vi "Retrieve Data.vi"(8 "error in (no error)":errorcluster, 11 "Vaisala in":refnum<class "FPGA Vaisala.lvclass">) -> (0 "error out":errorcluster, 2 "Str Out":string, 3 "Vaisala out":refnum<class "FPGA Vaisala.lvclass">)   [LabVIEW 2014, in "FPGA Vaisala.lvclass"]
uses:
  FPGA Vaisala.lvclass
  <vilib>/rvi/interface/nirviReadWriteControl/nirviReadWriteControl.xnode
  <vilib>/rvi/errors/niLvFpgaAdjustHostInterfaceError.vi
  Instruments/Nicholas/FPGA/RS485 In.ctl
  <vilib>/rvi/interface/nirviMethod/nirviMethod.xnode
  <vilib>/rvi/errors/niLvFpgaMergeErrorWithErrorCode.vi
  <vilib>/FPGAPlugInAG/cRIO-9081/niLvFpga_AcknowledgeIrq_cRIO-9081.vi
  <vilib>/rvi/interface/nirviMethod/StockFPGA_InlinedMethodWaitForSingleIRQ.vi
  <vilib>/FPGAPlugInAG/cRIO-9081/niLvFpga_WaitOnIrq_cRIO-9081.vi
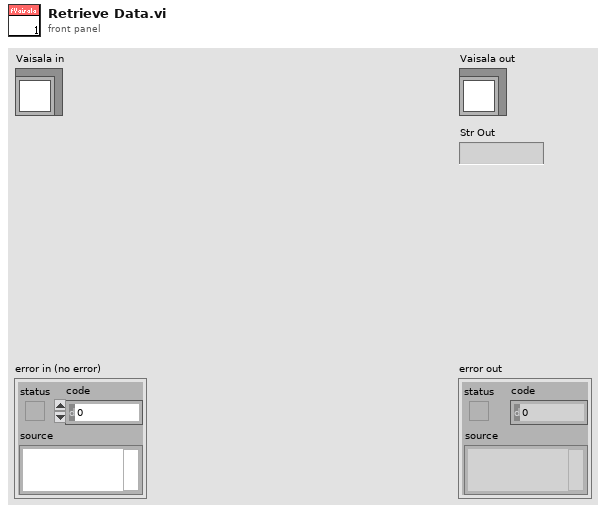
[diagram p1: front panel]
types:
  T1 = typedef "RS485 In.ctl" = cluster{"Data":u8[], "NumBytes":i32, "RS485_Cmd":enum16{"Read", "Write", "Idle"}, "New":bool, "Port":enum16{"Port 1", "Port 2", "Port 3", "Port 4", "None"}, "Timeout (ms)":i32}
  T2 = enum16{"Port 1", "Port 2", "Port 3", "Port 4", "None"}
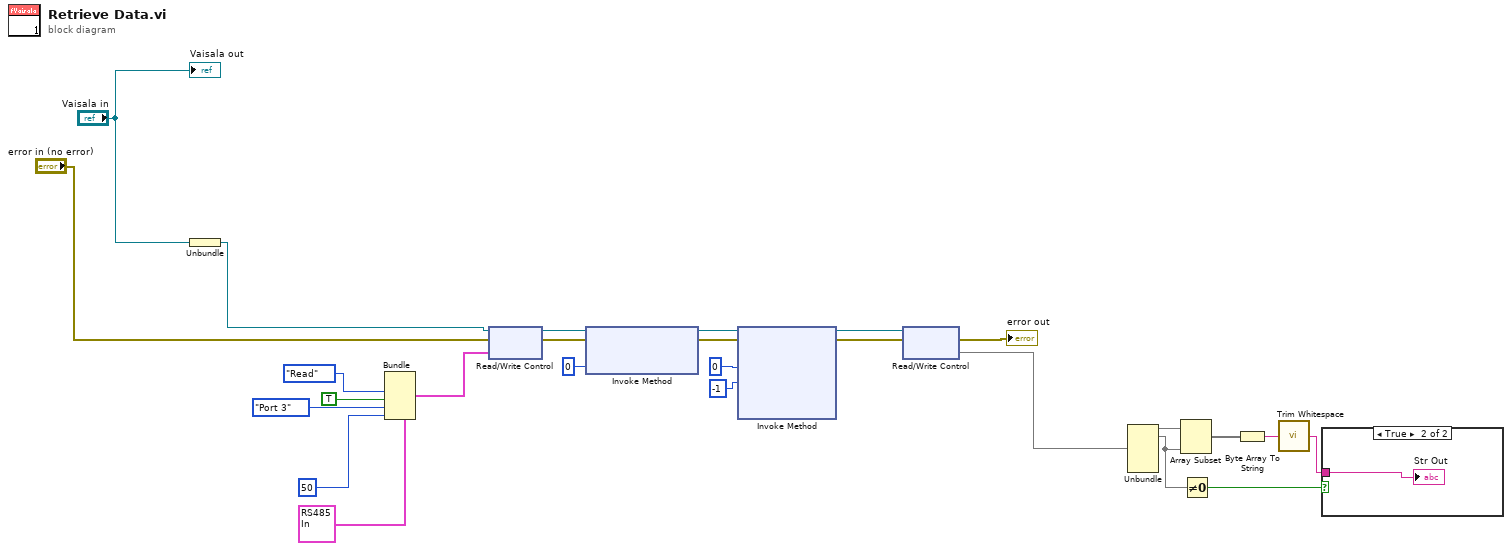
[diagram p0: block diagram]
diagram:
  n1 = Unbundle("Vaisala in") -> (w20:refnum<k20>)
  n2 = Bundle(cluster=T1 {"Data"=[0, 0, 0, 0, 0, 0, 0, 0, 0, 0, 0, 0, 0, 0, 0, 0, 0, 0, 0, 0, 0, 0, 0, 0, 0, 0, 0, 0, 0, 0, 0, 0, 0, 0, 0, 0, 0, 0, 0, 0, 0, 0, 0, 0, 0, 0, 0, 0, 0, 0, 0, 0, 0, 0, 0, 0, 0, 0, 0, 0, 0, 0, 0, 0, 0, 0, 0, 0, 0, 0, 0, 0, 0, 0, 0, 0, 0, 0, 0, 0, 0, 0, 0, 0, 0, 0, 0, 0, 0, 0, 0, 0, 0, 0, 0, 0, 0, 0, 0, 0], "NumBytes"=0, "RS485_Cmd"=enum."Write", "New"=FALSE, "Port"=enum."Port 1", "Timeout (ms)"=0} ("Input"), "RS485_Cmd"=enum16{"Read", "Write", "Idle"}."Read", "New"=TRUE ("New Message"), "Port"=T2."Port 3", "Timeout (ms)"=50) -> (w24:T1)  [unwired: 2 in]
  n3 = xnode "Read/Write Control"("FPGA VI Reference In"=w20, "error in"="error in (no error)", "Input"=w24) -> ("FPGA VI Reference Out"=w8:refnum<k20>, "error out"=w7:errorcluster)
  n4 = xnode "Invoke Method"("FPGA VI Reference In"=w8, "error in"=w7, "IRQ Number(s)"=0) -> ("FPGA VI Reference Out"=w12:refnum<k20>, "error out"=w11:errorcluster)
  n5 = xnode "Invoke Method"("FPGA VI Reference In"=w12, "error in"=w11, "IRQ Number(s)"=0, "Timeout (ms)"=-1) -> ("FPGA VI Reference Out"=w5:refnum<k20>, "error out"=w4:errorcluster)  [unwired: 2 out]
  n6 = xnode "Read/Write Control"("FPGA VI Reference In"=w5, "error in"=w4) -> ("error out"=→"error out":errorcluster, "Output"=w14)  [unwired: 1 out]
  n7 = Unbundle(w14) -> (w3, w2)  [unwired: 4 out]
  n8 = Array Subset(array=w3, length=w2) -> (w16:void[])  [unwired: 1 in]
  n9 = Not Equal To 0?(x=w2) -> (x != 0?=w15:bool)
  n10 = Byte Array To String(unsigned byte array=w16) -> (string=w18:string)
  n11 = call <vilib>:"Trim Whitespace.vi"("string"=w18) -> ("trimmed string"=w17:string)  [unwired: 1 in]
  n12 = case shown="True" w15 {
    tunnel: w17 -> [_ w27]
    frame False {
    }
    frame True {
      "Str Out" <- w27
    }
  }
  "Vaisala out" <- "Vaisala in"
